vi "Error_Logger.vi"(0 "Error_Log":bool caption="Error Log", 5 "Last_Error_Details":T1={"Error_Code"="", "Type"="Critical_Error", "Time"="27-01-2025 09:10:35", "Description"="Critical\nDevice Failure"} caption="Last Error Details") -> (4 "Error_Log_Table":string[][](array[string]))   [LabVIEW 2023]
doc: "Data logger used to log the data"
uses:
  Controls/Last_Error_Details.ctl
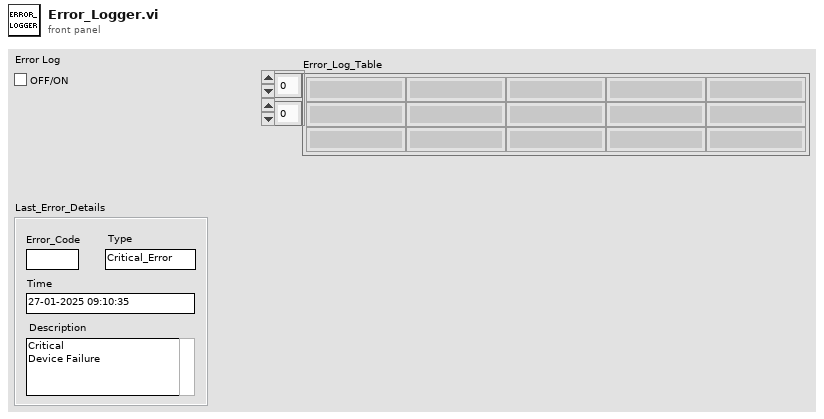
[diagram p1: front panel]
types:
  T1 = typedef "Last_Error_Details.ctl" = cluster{"Error_Code":string, "Type":string, "Time":string, "Description":string}
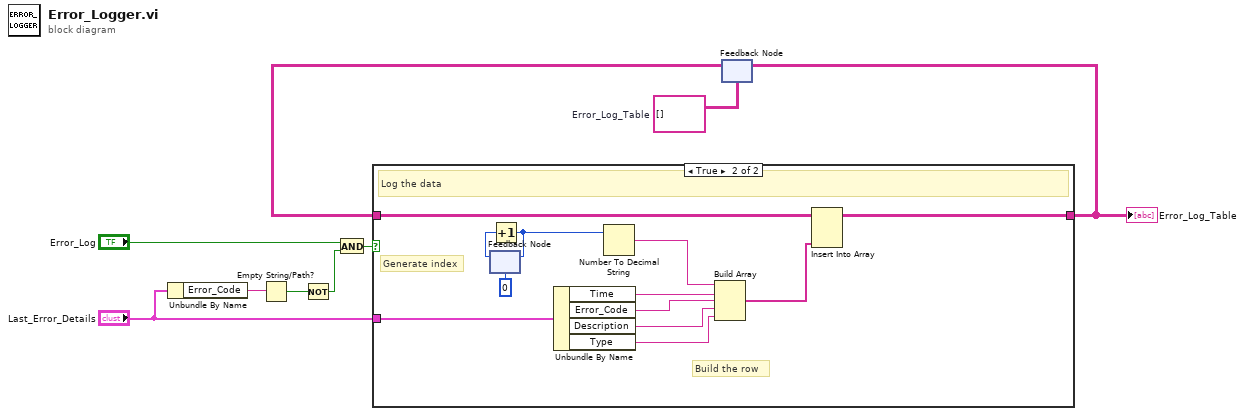
[diagram p0: block diagram]
diagram:
  w3 = string[][] []  # Error_Log_Table
  n1 = Unbundle By Name("Last_Error_Details") -> ("Error_Code"=w4:string)
  n2 = Empty String/Path?(string/path=w4) -> (empty?=w7:bool)
  n3 = Not(x=w7) -> (.not. x?=w6:bool)
  n4 = And(x="Error_Log", y=w6) -> (x .and. y?=w9:bool)
  n5 = feedback #1(w3) -> (w1:string[][])
  n6 = case shown="True" w9 {
    tunnel: "Last_Error_Details" -> [_ w16]
    tunnel: [w10 w14] -> w2
    tunnel: w1 -> [w10 w15]
    frame False {
      # "Dont Log"
    }
    frame True {
      # "Build the row"
      # "Generate index"
      # "Log the data"
      n7 = feedback #2(0) -> (w20:i32)
      n8 = Increment(x=w20) -> (x+1=w19:i32)
      n9 = feedback-in #2(w19) -> ()
      n10 = Unbundle By Name(w16) -> ("Time"=w12:string, "Error_Code"=w11:string, "Description"=w18:string, "Type"=w17:string)
      n11 = Number To Decimal String(number=w19) -> (decimal integer string=w22:string)  [unwired: 1 in]
      n12 = Build Array(w22, w12, w11, w18, w17) -> (w13:string[])
      n13 = Insert Into Array(array=w15, new element=w13) -> (w14:string[][])  [unwired: 2 in]
    }
  }
  "Error_Log_Table" <- w2
  n14 = feedback-in #1(w2) -> ()
